vi "Serial.vi"() -> ()   [LabVIEW 2025]
uses:
  <vilib>/Instr/_visa.llb/VISA Configure Serial Port (Instr).vi
panel:
  in  "Button":bool
  in  "write buffer":string
  in  "Stop":bool
  out "read buffer":string
  in  "VISA resource name":refnum<visa-resource-name>
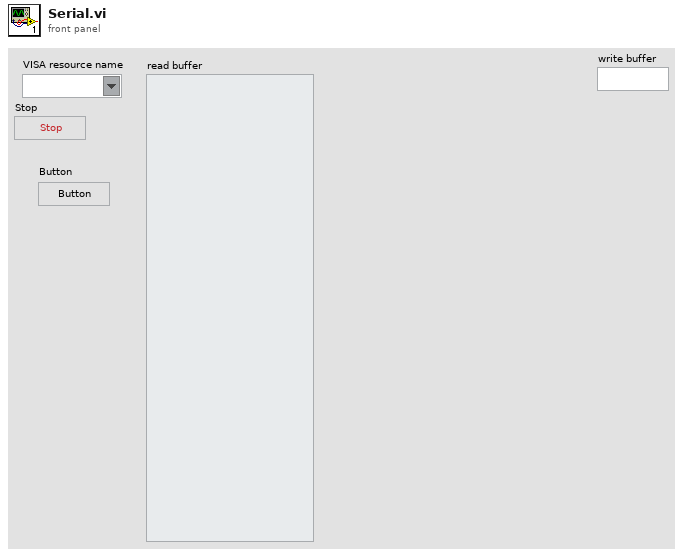
[diagram p1: front panel]
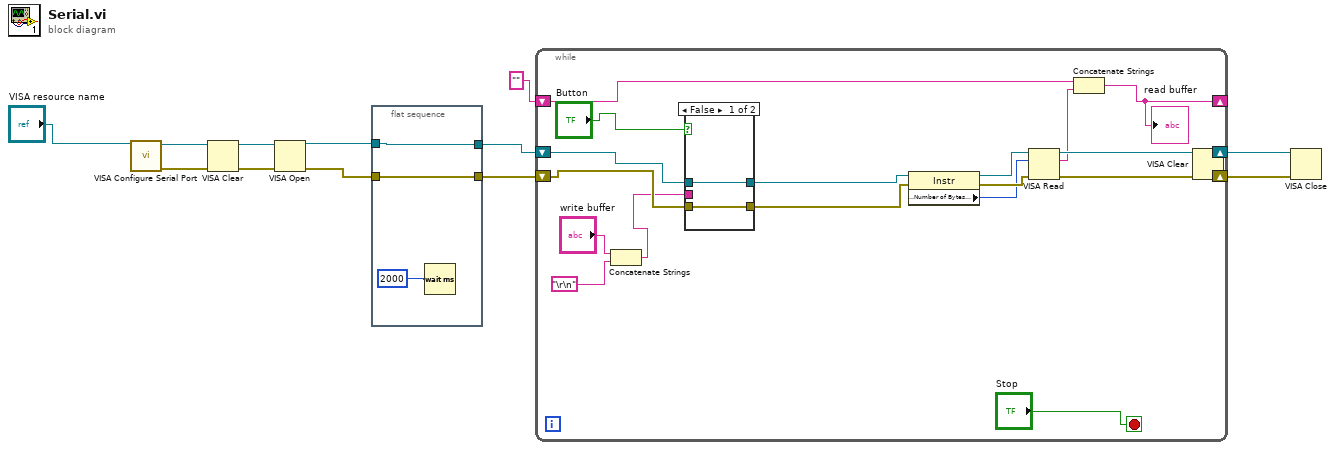
[diagram p0: block diagram]
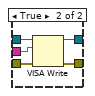
[diagram p2: hidden frame]
diagram:
  n1 = call-poly "VISA Configure Serial Port"("VISA resource name"="VISA resource name") -> ("VISA resource name out"=w2:refnum<visa-resource-name>, "error out"=w5:errorcluster)  [unwired: 13 in]
  n2 = VISA Clear(VISA resource name=w2, error in (no error)=w5) -> (VISA resource name out=w3:refnum<visa-resource-name>, error out=w4:errorcluster)
  n3 = VISA Open(error in (no error)=w4, VISA resource name=w3) -> (VISA resource name=w8:refnum<visa-resource-name>, error out=w7:errorcluster)  [unwired: 3 in]
  n4 = flat-sequence {
    tunnel: [w16] -> w9
    tunnel: w8 -> [w16]
    tunnel: [w15] -> w6
    tunnel: w7 -> [w15]
    frame #0 {
      n5 = Wait (ms)(milliseconds to wait=u32 2000) -> ()  [unwired: 1 out]
    }
  }
  n6 = while {
    shift-right: [w31] -> w10
    shift-left: w9 -> [w30]
    shift-right: [w32] -> w13
    shift-left: w6 -> [w29]
    shift-right: [w23] -> _
    shift-left: "" ("read buffer") -> [w25]
    stop <- "Stop" stop-if-true
    n7 = Concatenate Strings("write buffer", "\r\n") -> (w21:string)
    n8 = case shown="False" "Button" {
      tunnel: w21 -> [_ w41]
      tunnel: [w35 w40] -> w19
      tunnel: [w36 w39] -> w18
      tunnel: w30 -> [w35 w38]
      tunnel: w29 -> [w36 w37]
      frame False {
      }
      frame True {
        n9 = VISA Write(VISA resource name=w38, write buffer=w41, error in (no error)=w37) -> (VISA resource name out=w40:refnum<visa-resource-name>, error out=w39:errorcluster)  [unwired: 1 out]
      }
    }
    n10 = property class="Instr"(reference=w19, error in=w18) -> (reference out=w34:refnum<visa-resource-name>, error out=w33:errorcluster, "Serial Settings:Number of Bytes at Serial Port"=w28:u32)
    n11 = VISA Read(VISA resource name=w34, byte count=w28, error in (no error)=w33) -> (VISA resource name out=w31:refnum<visa-resource-name>, read buffer=w24:string, error out=w32:errorcluster)  [unwired: 1 out]
    n12 = Concatenate Strings(w25, w24) -> (w23:string)
    "read buffer" <- w23
  }
  n13 = VISA Clear(VISA resource name=w10, error in (no error)=w13) -> (VISA resource name out=w11:refnum<visa-resource-name>, error out=w12:errorcluster)
  n14 = VISA Close(VISA resource name=w11, error in (no error)=w12) -> ()  [unwired: 1 out]
